vi "SaveGraphDialog.vi"(8 "error (in)":errorcluster, 11 "reference (in)":refnum<vi>) -> (0 "error (out)":errorcluster, 3 "reference (out)":refnum<vi>)   [LabVIEW 2015]
panel:
  in  "OK Button":bool
  in  "Cancel Button":bool
  in  "Always Overwrite":bool
  in  "Hide Grid":bool
  in  "Target":enum32{"File", "Clipboard"}(ring)
  in  "File Type":enum32{"BMP", "EPS", "EMF", "PICT"}(ring)
  in  "File Path Control":path
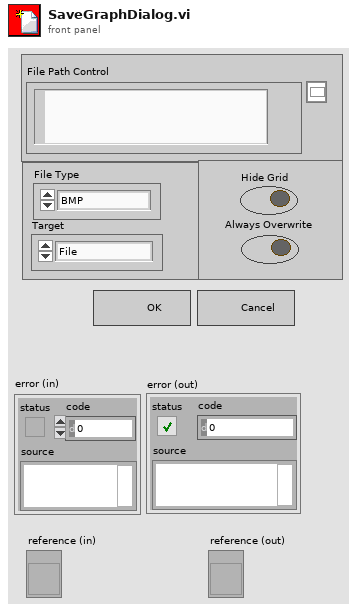
[diagram p1: front panel]
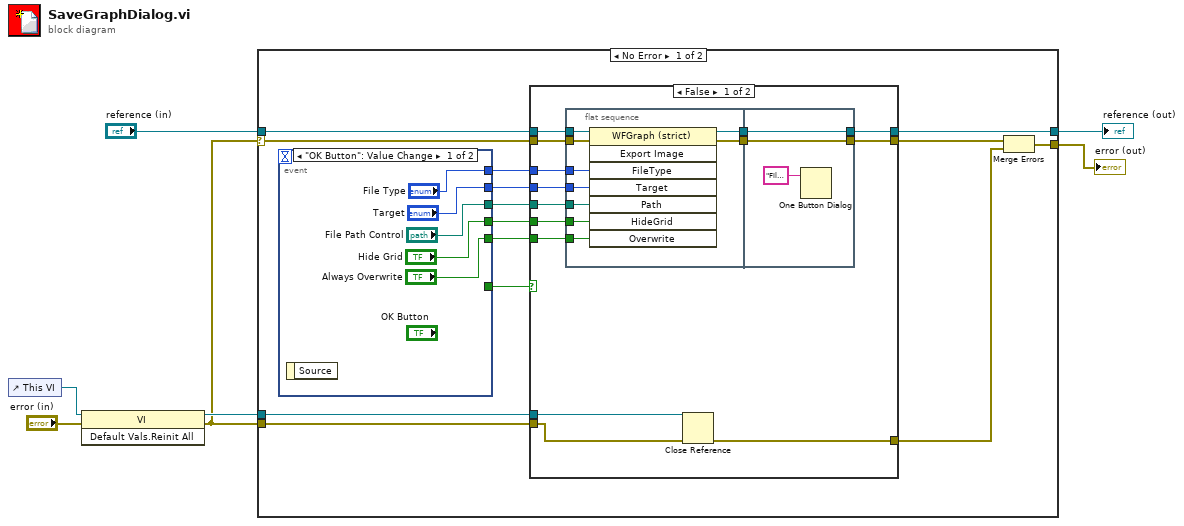
[diagram p0: block diagram]
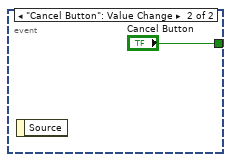
[diagram p2: hidden frame]
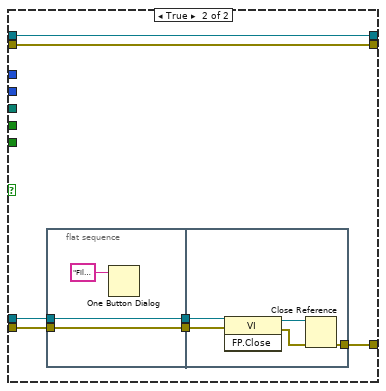
[diagram p3: hidden frame]
diagram:
  n1 = control-ref of="This VI"() -> (w6:refnum<vi>)
  n2 = invoke class="VI" method="Default Vals.Reinit All"(reference=w6, error in="error (in)") -> (reference out=w4:refnum<vi>, error out=w3:errorcluster)  [unwired: 1 in, 1 out]
  n3 = case shown="No Error" w3 {
    selector: w3 -> [w20 w69]
    tunnel: "reference (in)" -> [w21 w70]
    tunnel: [w9 w69] -> w7
    tunnel: [w19 w70] -> w1
    tunnel: w4 -> [w13 _]
    tunnel: w3 -> [w12 _]
    frame No Error {
      n4 = event shown="[0] \"OK Button\": Value Change" {
        selector: _ -> [_ _]
        dyn-events: _ -> [_ _]
        timeout: _ -> [_ _]
        tunnel: ["File Type" _] -> w18
        tunnel: ["Target" _] -> w17
        tunnel: ["File Path Control" _] -> w16
        tunnel: ["Hide Grid" _] -> w15
        tunnel: ["Always Overwrite" _] -> w14
        tunnel: [_ "Cancel Button"] -> w8
        event "OK Button": Value Change {
          n5 = event-data() -> ()  [unwired: 1 in, 1 out]
        }
        event "Cancel Button": Value Change {
          n6 = event-data() -> ()  [unwired: 1 in, 1 out]
        }
      }
      n7 = case shown="False" w8 {
        tunnel: w21 -> [w41 w57]
        tunnel: w20 -> [w40 w56]
        tunnel: [w39 w57] -> w19
        tunnel: [w38 w56] -> w10
        tunnel: w18 -> [w37 _]
        tunnel: w17 -> [w36 _]
        tunnel: w16 -> [w35 _]
        tunnel: w15 -> [w34 _]
        tunnel: w14 -> [w33 _]
        tunnel: w13 -> [w30 w60]
        tunnel: w12 -> [w29 w59]
        tunnel: [w28 w58] -> w11
        frame False {
          n8 = flat-sequence {
            tunnel: w41 -> [w50]
            tunnel: w40 -> [w49]
            tunnel: w37 -> [w46]
            tunnel: w36 -> [w45]
            tunnel: w35 -> [w44]
            tunnel: w34 -> [w43]
            tunnel: w33 -> [w42]
            tunnel: [w48] -> w32
            tunnel: [w47] -> w31
            tunnel: [w52] -> w38
            tunnel: [w53] -> w39
            tunnel: w32 -> [w53]
            tunnel: w31 -> [w52]
            frame #0 {
              n9 = invoke on="Invoke Node" class="WFGraph (strict)" method="Export Image"(reference=w50, error in=w49, "FileType"=w46, "Target"=w45, "Path"=w44, "HideGrid"=w43, "Overwrite"=w42) -> (reference out=w48:refnum<vi>, error out=w47:errorcluster)  [unwired: 1 in, 6 out]
            }
            frame #1 {
              n10 = One Button Dialog(message="File successfully saved!") -> ()  [unwired: 1 in, 1 out]
            }
          }
          n11 = Close Reference(reference=w30, error in (no error)=w29) -> (error out=w28:errorcluster)
        }
        frame True {
          n12 = flat-sequence {
            tunnel: w59 -> [w62]
            tunnel: w60 -> [w63]
            tunnel: [w63] -> w55
            tunnel: [w62] -> w54
            tunnel: [w64] -> w58
            tunnel: w55 -> [w66]
            tunnel: w54 -> [w65]
            frame #0 {
              n13 = One Button Dialog(message="File save has been cancelled!") -> ()  [unwired: 1 in, 1 out]
            }
            frame #1 {
              n14 = invoke class="VI" method="FP.Close"(reference=w66, error in=w65) -> (reference out=w68:refnum<vi>, error out=w67:errorcluster)  [unwired: 1 in, 1 out]
              n15 = Close Reference(reference=w68, error in (no error)=w67) -> (error out=w64:errorcluster)
            }
          }
        }
      }
      n16 = Merge Errors(w10, w11) -> (w9:errorcluster)
    }
    frame Error {
    }
  }
  "error (out)" <- w7
  "reference (out)" <- w1
